vi "USB4000_ACQ.vi"(8 "error in (no error)":errorcluster, 10 "Type":enum16{"Get Background", "Measure", "Raw"}(ring)=enum."Measure", 11 "Instruments in":refnum<class "Instruments.lvclass">) -> (0 "error out":errorcluster, 2 "Peak Wl":dbl, 3 "Instruments out":refnum<class "Instruments.lvclass">)   [LabVIEW 2012, in "Instruments.lvclass"]
uses:
  Instruments.lvclass
  Instruments.lvclass/Instruments.ctl
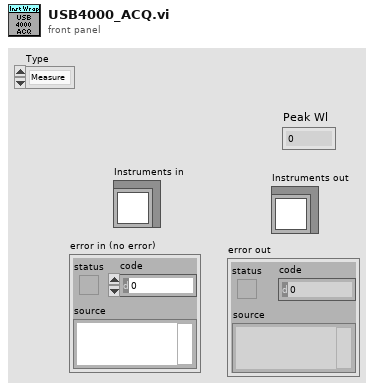
[diagram p1: front panel]
types:
  T1 = typedef "USB4000_Data.ctl" = cluster{"Wrapper Out":u32, "Number of Spectrometers":i32, "Wavelength":dbl[], "EL Spectrum":dbl[], "Int Time (usec)":i32, bool, "Background":dbl[]}
  T2 = typedef "Config.ctl" = cluster{"IntTime":i32, "Samples":i32, "PowerMin":dbl, "KneeMin":dbl, "KneeMax":dbl, "BackgroundWl":dbl}
  T3 = cluster{"Keithley_Param":cluster{"Start Current,mA":dbl, "Stop Current,mA":dbl, "Voltage Compliance,V":dbl, "GPIB":string}, "USB4000_Param":cluster{"Integration Time":i32, "Wl min,nm":dbl, "Wl max,nm":dbl, "USB4000":T1}, "Ophir_Param":cluster{"VISA resource name":refnum<visa-resource-name>, "Calibration Wl":dbl}, "Config":T2}
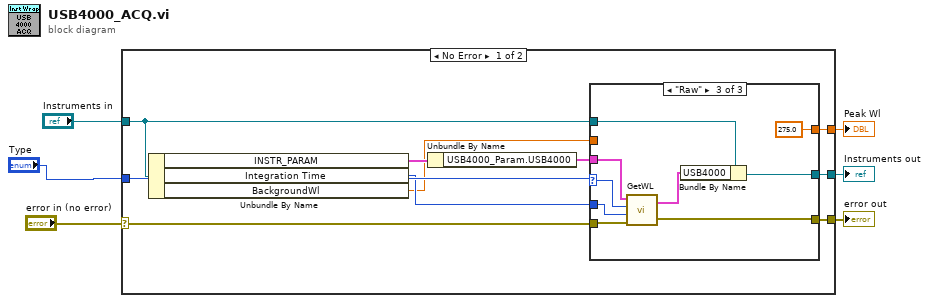
[diagram p0: block diagram]
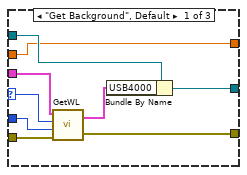
[diagram p2: hidden frame]
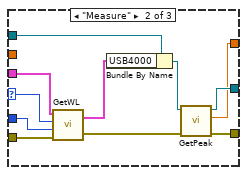
[diagram p3: hidden frame]
diagram:
  n1 = case shown="No Error" "error in (no error)" {
    selector: "error in (no error)" -> [w9 w47]
    tunnel: [w11 w47] -> w5
    tunnel: [w12 w46] -> w3
    tunnel: "Instruments in" -> [w13 w46]
    tunnel: "Type" -> [w16 _]
    tunnel: [w15 _] -> w2
    frame No Error {
      n2 = Unbundle By Name(w13) -> ("INSTR_PARAM"=w14:T3, "Integration Time"=w8:i32, "BackgroundWl"=w7:dbl)
      n3 = Unbundle By Name(w14) -> ("USB4000_Param.USB4000"=w10:T1)
      n4 = case shown="\"Raw\"" w16 {
        selector: w16 -> [w24 w26 w40]
        tunnel: w10 -> [w25 w28 w42]
        tunnel: w9 -> [w23 w29 w41]
        tunnel: w13 -> [w21 w36 w43]
        tunnel: [w19 w33 w44] -> w12
        tunnel: [w22 w31 w38] -> w11
        tunnel: [w17 w32 275.0 ("Peak Wl")] -> w15
        tunnel: w8 -> [w18 w27 w39]
        tunnel: w7 -> [w17 _ _]
        frame "Get Background", Default {
          n5 = call "GetWL.vi"("error in (no error)"=w23, "Integration Time"=w18, "Type"=w24, "USB4000 Params In"=w25) -> ("error out"=w22:errorcluster, "USB4000 Params Out"=w20:T1)
          n6 = Bundle By Name(cluster=w21, "USB4000"=w20) -> (w19:refnum<class "Instruments.lvclass">)
        }
        frame "Measure" {
          n7 = call "GetWL.vi"("error in (no error)"=w29, "Integration Time"=w27, "Type"=w26, "USB4000 Params In"=w28) -> ("error out"=w30:errorcluster, "USB4000 Params Out"=w35:T1)
          n8 = Bundle By Name(cluster=w36, "USB4000"=w35) -> (w34:refnum<class "Instruments.lvclass">)
          n9 = call-dynamic "GetPeak.vi"("error in (no error)"=w30, "Instruments in"=w34) -> ("error out"=w31:errorcluster, "Peak Wl"=w32:dbl, "Instruments out"=w33:refnum<class "Instruments.lvclass">)  [unwired: 7 in]
        }
        frame "Raw" {
          n10 = call "GetWL.vi"("error in (no error)"=w41, "Integration Time"=w39, "Type"=w40, "USB4000 Params In"=w42) -> ("error out"=w38:errorcluster, "USB4000 Params Out"=w45:T1)
          n11 = Bundle By Name(cluster=w43, "USB4000"=w45) -> (w44:refnum<class "Instruments.lvclass">)
        }
      }
    }
    frame Error {
    }
  }
  "error out" <- w5
  "Instruments out" <- w3
  "Peak Wl" <- w2
